vi "Release Lock from Alarm.vi"(11 "error in (no error)":errorcluster) -> (15 "error out":errorcluster)   [LabVIEW 2024, in "GRBL 1.1.lvlib"]
doc: "Overside Alarm lock to allow for Axis movement."
uses:
  GRBL 1.1.lvlib
panel:
  out "Data read":string
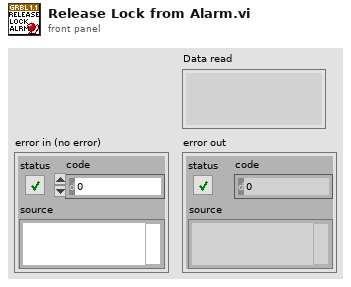
[diagram p1: front panel]
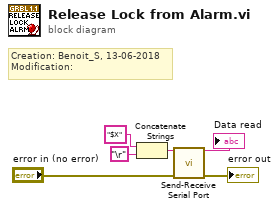
[diagram p0: block diagram]
diagram:
  # "Creation: Benoit_S, 13-06-2018\nModification:"
  n1 = Concatenate Strings("$X" ("Data to write"), "\r") -> (w3:string)
  n2 = call "Send-Receive Serial Port.vi"("Data to write"=w3, "error in (no error)"="error in (no error)") -> ("Data read"=→"Data read":string, "error out"=→"error out":errorcluster)  [unwired: 12 in]
